vi "DAQmx.Activity Tree.vi"(8 "error in (no error)":errorcluster, 11 "Refnum in":refnum<k21>) -> ()   [LabVIEW 2019, in "Instrument.DAQ.lvclass"]
uses:
  Instrument.DAQ.lvclass
  <resource>/objmgr/daqmx.rc
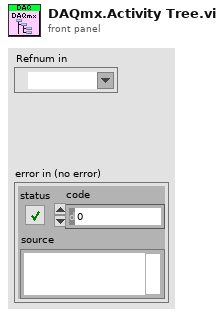
[diagram p1: front panel]
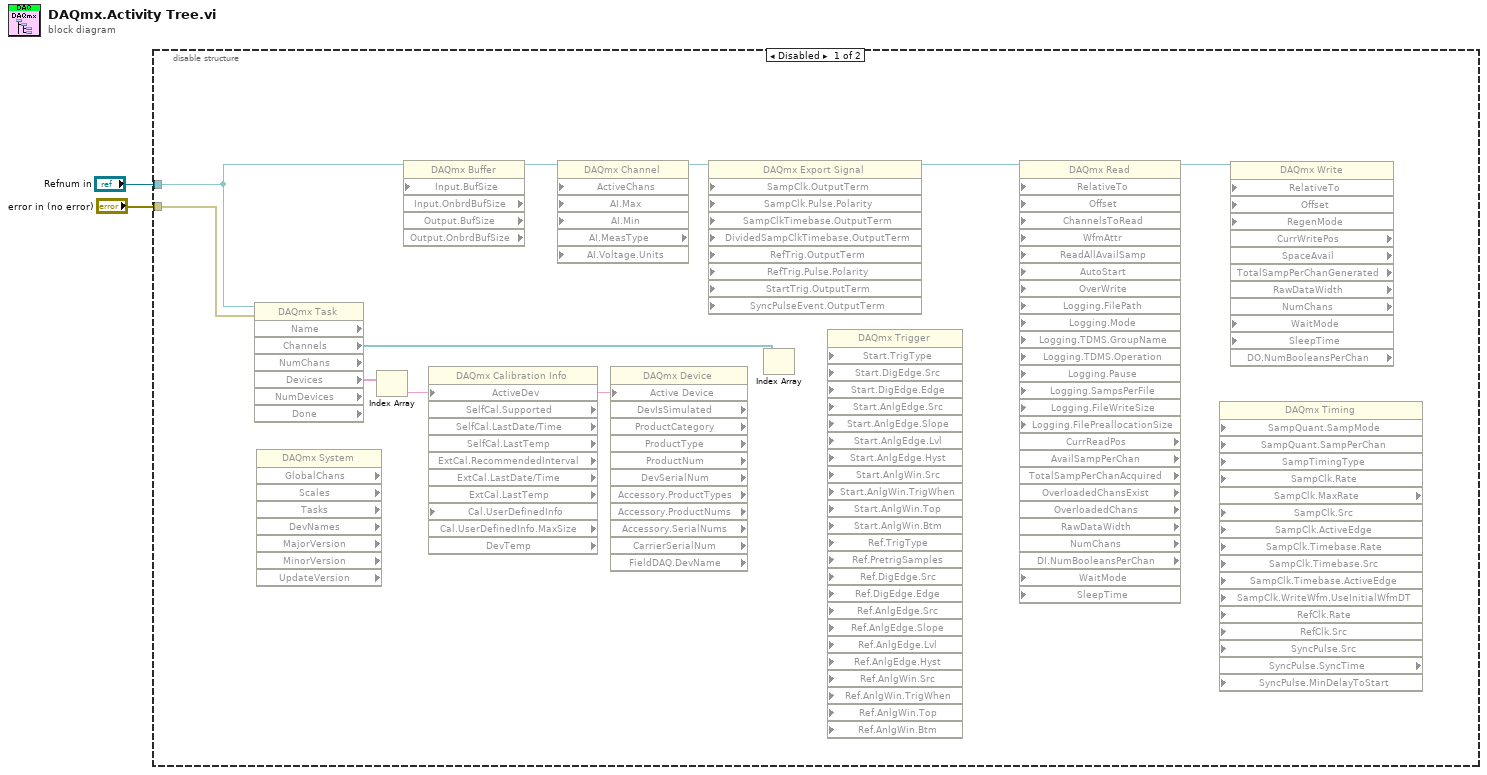
[diagram p0: block diagram]
diagram:
  n1 = disable-structure shown="Disabled" {
    disable-tunnel: "error in (no error)" -> [w11 _]
    disable-tunnel: "Refnum in" -> [w9 _]
    frame Disabled {
      n2 = property class="DAQmx Task" props=["Name", "Channels", "NumChans", "Devices", "NumDevices", "Done"](reference=w9, error in=w11) -> ("Channels"=w5:refnum<k21>[], "Devices"=w10:tag[])  [unwired: 6 out]
      n3 = property class="DAQmx System" props=["GlobalChans", "Scales", "Tasks", "DevNames", "MajorVersion", "MinorVersion", "UpdateVersion"]() -> ()  [unwired: 2 in, 9 out]
      n4 = Index Array(array=w10) -> (element=w6:tag)  [unwired: 1 in]
      n5 = property class="DAQmx Buffer" props=["Input.BufSize", "Input.OnbrdBufSize", "Output.BufSize", "Output.OnbrdBufSize"](reference=w9) -> (reference out=w7:refnum<k21>)  [unwired: 2 in, 4 out]
      n6 = property class="DAQmx Calibration Info" props=["ActiveDev", "SelfCal.Supported", "SelfCal.LastDate/Time", "SelfCal.LastTemp", "ExtCal.RecommendedInterval", "ExtCal.LastDate/Time", "ExtCal.LastTemp", "Cal.UserDefinedInfo", "Cal.UserDefinedInfo.MaxSize", "DevTemp"]("ActiveDev"=w6) -> ()  [unwired: 3 in, 10 out]
      n7 = property class="DAQmx Channel" props=["ActiveChans", "AI.Max", "AI.Min", "AI.MeasType", "AI.Voltage.Units"](reference=w7) -> (reference out=w8:refnum<k21>)  [unwired: 5 in, 2 out]
      n8 = property class="DAQmx Device" props=["Active Device", "DevIsSimulated", "ProductCategory", "ProductType", "ProductNum", "DevSerialNum", "Accessory.ProductTypes", "Accessory.ProductNums", "Accessory.SerialNums", "CarrierSerialNum", "FieldDAQ.DevName"]("Active Device"=w6) -> ()  [unwired: 2 in, 12 out]
      n9 = property class="DAQmx Export Signal" props=["SampClk.OutputTerm", "SampClk.Pulse.Polarity", "SampClkTimebase.OutputTerm", "DividedSampClkTimebase.OutputTerm", "RefTrig.OutputTerm", "RefTrig.Pulse.Polarity", "StartTrig.OutputTerm", "SyncPulseEvent.OutputTerm"](reference=w8) -> (reference out=w4:refnum<k21>)  [unwired: 9 in, 1 out]
      n10 = Index Array(array=w5) -> ()  [unwired: 1 in, 1 out]
      n11 = property class="DAQmx Trigger" props=["Start.TrigType", "Start.DigEdge.Src", "Start.DigEdge.Edge", "Start.AnlgEdge.Src", "Start.AnlgEdge.Slope", "Start.AnlgEdge.Lvl", "Start.AnlgEdge.Hyst", "Start.AnlgWin.Src", "Start.AnlgWin.TrigWhen", "Start.AnlgWin.Top", "Start.AnlgWin.Btm", "Ref.TrigType", "Ref.PretrigSamples", "Ref.DigEdge.Src", "Ref.DigEdge.Edge", "Ref.AnlgEdge.Src", "Ref.AnlgEdge.Slope", "Ref.AnlgEdge.Lvl", "Ref.AnlgEdge.Hyst", "Ref.AnlgWin.Src", "Ref.AnlgWin.TrigWhen", "Ref.AnlgWin.Top", "Ref.AnlgWin.Btm"]() -> ()  [unwired: 25 in, 2 out]
      n12 = property class="DAQmx Read" props=["RelativeTo", "Offset", "ChannelsToRead", "WfmAttr", "ReadAllAvailSamp", "AutoStart", "OverWrite", "Logging.FilePath", "Logging.Mode", "Logging.TDMS.GroupName", "Logging.TDMS.Operation", "Logging.Pause", "Logging.SampsPerFile", "Logging.FileWriteSize", "Logging.FilePreallocationSize", "CurrReadPos", "AvailSampPerChan", "TotalSampPerChanAcquired", "OverloadedChansExist", "OverloadedChans", "RawDataWidth", "NumChans", "DI.NumBooleansPerChan", "WaitMode", "SleepTime"](reference=w4) -> (reference out=w3:refnum<k21>)  [unwired: 18 in, 9 out]
      n13 = property class="DAQmx Timing" props=["SampQuant.SampMode", "SampQuant.SampPerChan", "SampTimingType", "SampClk.Rate", "SampClk.MaxRate", "SampClk.Src", "SampClk.ActiveEdge", "SampClk.Timebase.Rate", "SampClk.Timebase.Src", "SampClk.Timebase.ActiveEdge", "SampClk.WriteWfm.UseInitialWfmDT", "RefClk.Rate", "RefClk.Src", "SyncPulse.Src", "SyncPulse.SyncTime", "SyncPulse.MinDelayToStart"]() -> ()  [unwired: 16 in, 4 out]
      n14 = property class="DAQmx Write" props=["RelativeTo", "Offset", "RegenMode", "CurrWritePos", "SpaceAvail", "TotalSampPerChanGenerated", "RawDataWidth", "NumChans", "WaitMode", "SleepTime", "DO.NumBooleansPerChan"](reference=w3) -> ()  [unwired: 6 in, 8 out]
    }
    frame Enabled {
    }
  }
